vi "Read Command Options.vi"(8 "error in (no error)":errorcluster, 11 "Console Wrapper in":refnum<class "Console Wrapper.lvclass">) -> (0 "error out":errorcluster, 2 "Command Options":string, 3 "Console Wrapper out":refnum<class "Console Wrapper.lvclass">)   [LabVIEW 2020, in "Console Wrapper.lvclass"]
uses:
  Console Wrapper.lvclass
  Console Wrapper.lvclass/Console Wrapper.ctl
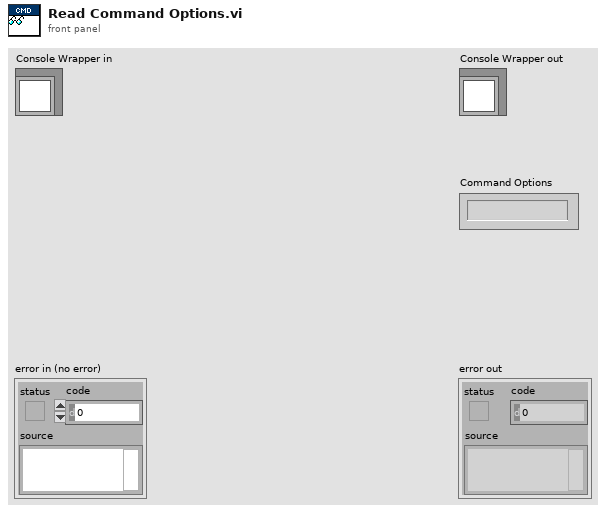
[diagram p1: front panel]
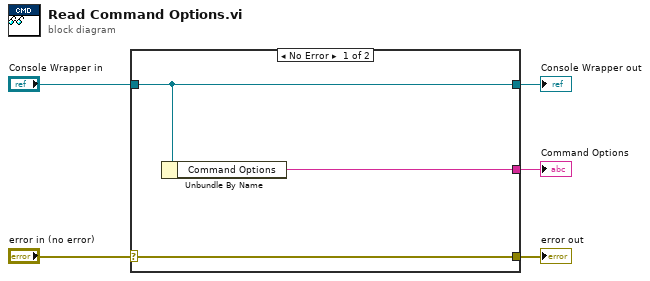
[diagram p0: block diagram]
diagram:
  n1 = case shown="No Error" "error in (no error)" {
    selector: "error in (no error)" -> [w8 w9]
    tunnel: [w8 w9] -> w4
    tunnel: [w7 w10] -> w2
    tunnel: "Console Wrapper in" -> [w7 w10]
    tunnel: [w6 _] -> w1
    frame No Error {
      n2 = Unbundle By Name(w7) -> ("Command Options"=w6:string)
    }
    frame Error {
    }
  }
  "error out" <- w4
  "Console Wrapper out" <- w2
  "Command Options" <- w1
